vi "Close Moxa_2.vi"(8 "error in (no error)":errorcluster) -> (0 "error out":errorcluster)   [LabVIEW 2022 SP3]
doc: "Closes Moxa device"
uses:
  <vilib>/NI/Modbus Library/API/Master/Modbus Master.lvclass
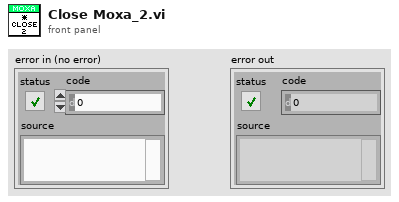
[diagram p1: front panel]
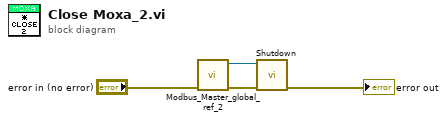
[diagram p0: block diagram]
diagram:
  n1 = call "Modbus_Master_global_ref_2.vi"("error in (no error) 2"="error in (no error)") -> ("error out 2"=w2:errorcluster, "Modbus Master out"=w1:refnum<class "Modbus Master.lvclass">)  [unwired: 9 in]
  n2 = call-dynamic "Shutdown.vi"("error in"=w2, "Modbus master in"=w1) -> ("error out"=→"error out":errorcluster)  [unwired: 9 in]
